vi "Counter read.vi"(7 "IP":string="192.168.23.100", 8 "error in (no error)":errorcluster, 9 "Select Counter":i8=1 min=1 max=2 step=1, 10 "PORT":dbl=1.0 min=1.0 max=4.0 step=1.0, 11 "MASTER":dbl=1.0 min=1.0 max=10.0 step=1.0) -> (0 "error out":errorcluster, 3 "COUNTER":u32 format="%^#.10g")   [LabVIEW 2022 SP3]
uses:
  <vilib>/JDP Science/JSONtext/JSONtext.lvlib
panel:
  out "JSON DATA":string
  # "Counter reader"
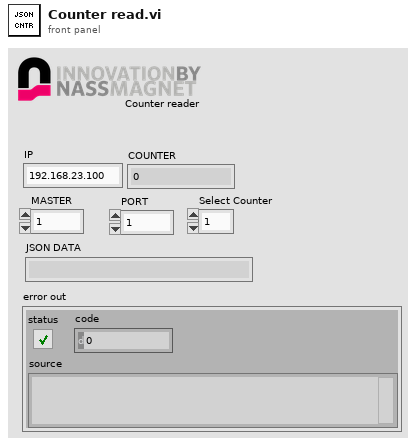
[diagram p1: front panel]
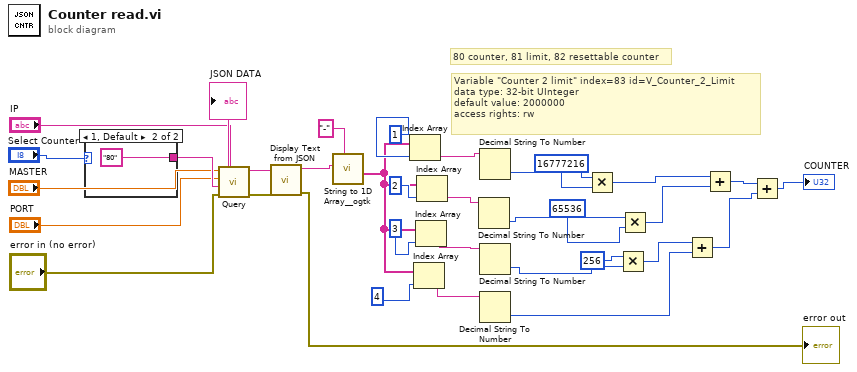
[diagram p0: block diagram]
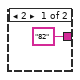
[diagram p2: hidden frame]
diagram:
  # "Variable \"Counter 2 limit\" index=83 id=V_Counter_2_Limit\ndata type: 32-bit UInteger\ndefault value: 2000000\naccess rights: rw"
  # "80 counter, 81 limit, 82 resettable counter"
  n1 = case shown="1, Default" "Select Counter" {
    tunnel: ["82" ("PARAMETERS") "80" ("PARAMETERS")] -> w23
    frame 2 {
    }
    frame 1, Default {
    }
  }
  n2 = call "Query.vi"("IP"="IP", "error in (no error)"="error in (no error)", "PARAMETERS"=w23, "PORT"="PORT", "MASTER"="MASTER") -> ("error out"=w20:errorcluster, "Response"=w33:string)  [unwired: 5 in]
  "JSON DATA" <- w33
  n3 = call <vilib>:"Display Text from JSON.vi"("error in (no error)"=w20, "Input JSON"=w33) -> ("error out"=→"error out":errorcluster, "Display Text"=w9:string)  [unwired: 7 in, 1 out]
  n4 = call <userlib>:"String to 1D Array__ogtk.vi"("delimiter (Tab)"="-", "string"=w9) -> ("Array of Strings"=w26:string[])  [unwired: 9 in]
  n5 = Index Array(array=w26, index=1) -> (element=w10:string)
  n6 = Index Array(array=w26, index=4) -> (element=w13:string)
  n7 = Index Array(array=w26, index=3) -> (element=w12:string)
  n8 = Index Array(array=w26, index=2) -> (element=w11:string)
  n9 = Decimal String To Number(string=w11) -> (number=w17:i32)  [unwired: 2 in, 1 out]
  n10 = Decimal String To Number(string=w10) -> (number=w6:i32)  [unwired: 2 in, 1 out]
  n11 = Decimal String To Number(string=w12) -> (number=w2:i32)  [unwired: 2 in, 1 out]
  n12 = Decimal String To Number(string=w13) -> (number=w8:i32)  [unwired: 2 in, 1 out]
  n13 = Multiply(x=w6, y=u32 16777216) -> (x*y=w7:u32)
  n14 = Multiply(x=u32 256 ("y"), y=w2) -> (x*y=w15:u32)
  n15 = Multiply(x=w17, y=u32 65536) -> (x*y=w14:u32)
  n16 = Add(x=w15, y=w8) -> (x+y=w24:u32)
  n17 = Add(x=w7, y=w14) -> (x+y=w25:u32)
  n18 = Add(x=w25, y=w24) -> (x+y=→"COUNTER":u32)
